vi "Configure Queue Connection.vi"(6 "timeout (500 ms)":i32=500, 8 "error in (no error)":errorcluster, 11 "Queue Name":string) -> (0 "error out":errorcluster, 3 "LocalQueueConnection":refnum<class "LocalQueueConnection.lvclass">)   [LabVIEW 2013, in "MQTT_Queue.lvlib" / "LocalQueueConnection.lvclass"]
uses:
  LocalQueueConnection.lvclass
  <vilib>/LabVIEW Open Source Project/Connection/Connection/Connection.lvclass/Connection.ctl
  LocalQueueConnection.lvclass/LocalQueueConnection.ctl
  <vilib>/LabVIEW Open Source Project/Connection/Connection/Connection.lvclass
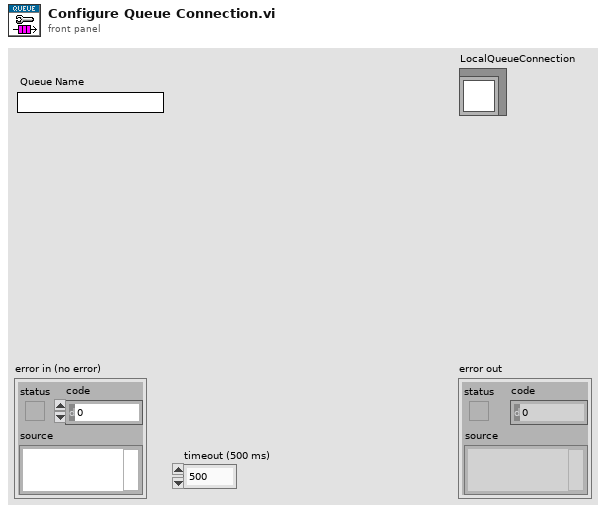
[diagram p1: front panel]
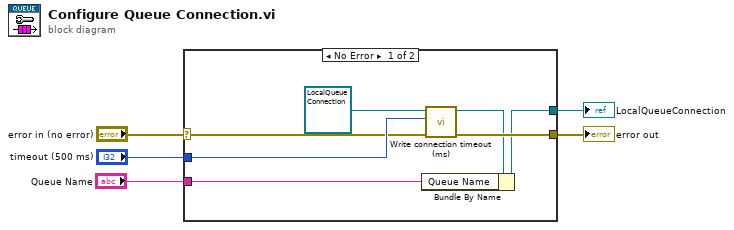
[diagram p0: block diagram]
diagram:
  n1 = case shown="No Error" "error in (no error)" {
    selector: "error in (no error)" -> [w11 w13]
    tunnel: [w10 w13] -> w4
    tunnel: [w7 _] -> w2
    tunnel: "timeout (500 ms)" -> [w12 _]
    tunnel: "Queue Name" -> [w6 _]
    frame No Error {
      n2 = call <vilib>:"Write connection timeout (ms).vi"("error in (no error)"=w11, "connection timeout (ms)"=w12, "Connection in"=refnum<class "LocalQueueConnection.lvclass"> refnum ("TCPConnection in")) -> ("error out"=w10:errorcluster, "Connection out"=w8:refnum<class "LocalQueueConnection.lvclass">)  [unwired: 7 in]
      n3 = Bundle By Name(cluster=w8, "Queue Name"=w6) -> (w7:refnum<class "LocalQueueConnection.lvclass">)
    }
    frame Error {
    }
  }
  "error out" <- w4
  "LocalQueueConnection" <- w2
